vi "EnqueuePoint.vi"(0 "queue in":T1, 5 "channel":string, 7 "time":timestamp, 9 "value":dbl, 11 "error in (no error)":errorcluster) -> (4 "queue out":T1, 6 "# elements in queue":i32, 15 "error out":errorcluster)   [LabVIEW 2022 SP3]
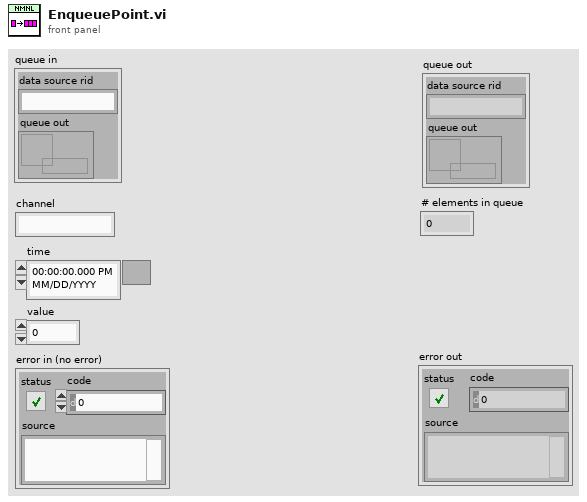
[diagram p1: front panel]
types:
  T1 = cluster{"data source rid":string, "queue out":refnum<queue>}
  T2 = cluster{"channel":string, "time_seconds":i32, "time_nanos":i32, "value":dbl}
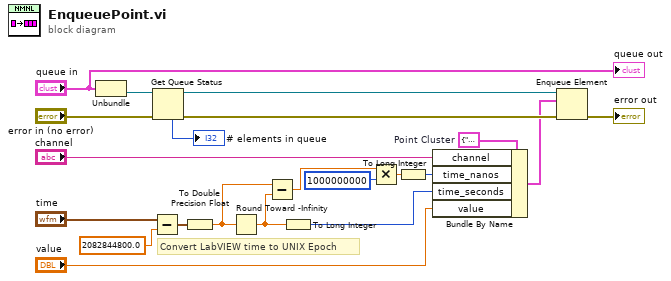
[diagram p0: block diagram]
diagram:
  w7 = T2 {"channel"="", "time_seconds"=0, "time_nanos"=0, "value"=0.0}  # Point Cluster
  # "Convert LabVIEW time to UNIX Epoch"
  n1 = Unbundle("queue in") -> ("queue out"=w4:refnum<queue>)  [unwired: 1 out]
  n2 = Subtract(x="time", y=2082844800.0) -> (x-y=w19:timestamp)
  n3 = Get Queue Status(queue=w4, error in (no error)="error in (no error)") -> (queue out=w21:refnum<queue>, error out=w20:errorcluster, # elements in queue=→"# elements in queue":i32)  [unwired: 1 in, 5 out]
  n4 = To Double Precision Float(number=w19) -> (double precision float=w16:dbl)
  n5 = Round Toward -Infinity(1:w16) -> (0:w15:dbl)
  n6 = Subtract(x=w16, y=w15) -> (x-y=w3:dbl)
  n7 = To Long Integer(number=w15) -> (32bit integer=w17:i32)
  n8 = Multiply(x=w3, y=u32 1000000000) -> (x*y=w2:dbl)
  n9 = To Long Integer(number=w2) -> (32bit integer=w1:i32)
  n10 = Bundle By Name(cluster=w7, "channel"="channel", "time_nanos"=w1, "time_seconds"=w17, "value"="value") -> (w6:T2)
  n11 = Enqueue Element(queue=w21, element=w6, error in (no error)=w20) -> (error out=→"error out":errorcluster)  [unwired: 1 in, 2 out]
  "queue out" <- "queue in"
